vi "op_biti_v1_02.vi"() -> ()   [LabVIEW 2009]
uses:
  <vilib>/Platform/portaccess.llb/Out Port8.vi
panel:
  in  "Numeric":u8=75
  out "Array":bool[](array[boolean])=[FALSE, TRUE, FALSE, FALSE, TRUE, FALSE, TRUE, TRUE]
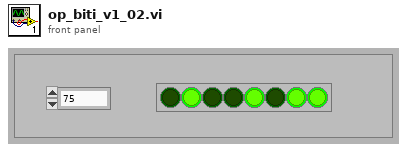
[diagram p1: front panel]
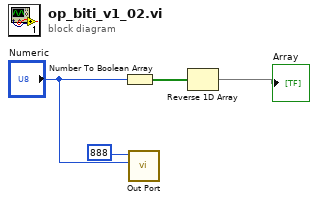
[diagram p0: block diagram]
diagram:
  n1 = Number To Boolean Array(number="Numeric") -> (Boolean array=w4:bool[])
  n2 = call-poly <vilib>:"Out Port.vi"("write value"="Numeric", "address"=888) -> ()  [unwired: 7 in, 1 out]
  n3 = Reverse 1D Array(array=w4) -> (reversed array=→"Array":bool[])
